vi "LV SciSDK INIT TOF SPECTRUM.vi"(0 "TOF Spectrum Name":string, 5 "Bin Width":u32, 7 "Start Delay":u32, 9 "Handle In":T2, 11 "error in (no error)":errorcluster) -> (10 "TOF Spectrum Handle Out":T1, 15 "error out":errorcluster)   [LabVIEW 2021]
uses:
  SciSDK_Labview.lvlib
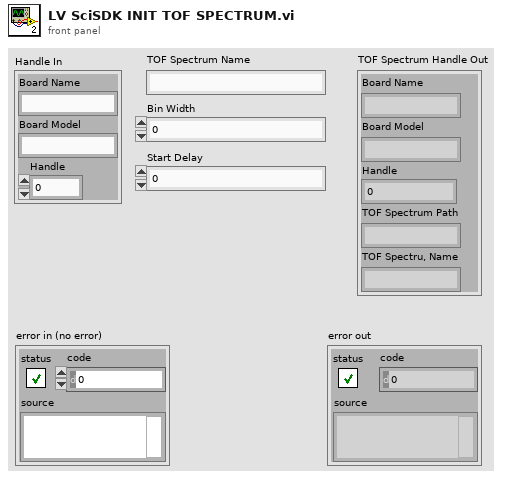
[diagram p1: front panel]
types:
  T1 = cluster{"Board Name":string, "Board Model":string, "Handle":u64, "TOF Spectrum Path":string, "TOF Spectru, Name":string}
  T2 = cluster{"Board Name":string, "Board Model":string, "Handle":u64}
  T3 = cluster{"Board Name":string, "Board Model":string, "Handle":u64, string, "TOF Spectrum Name":string}
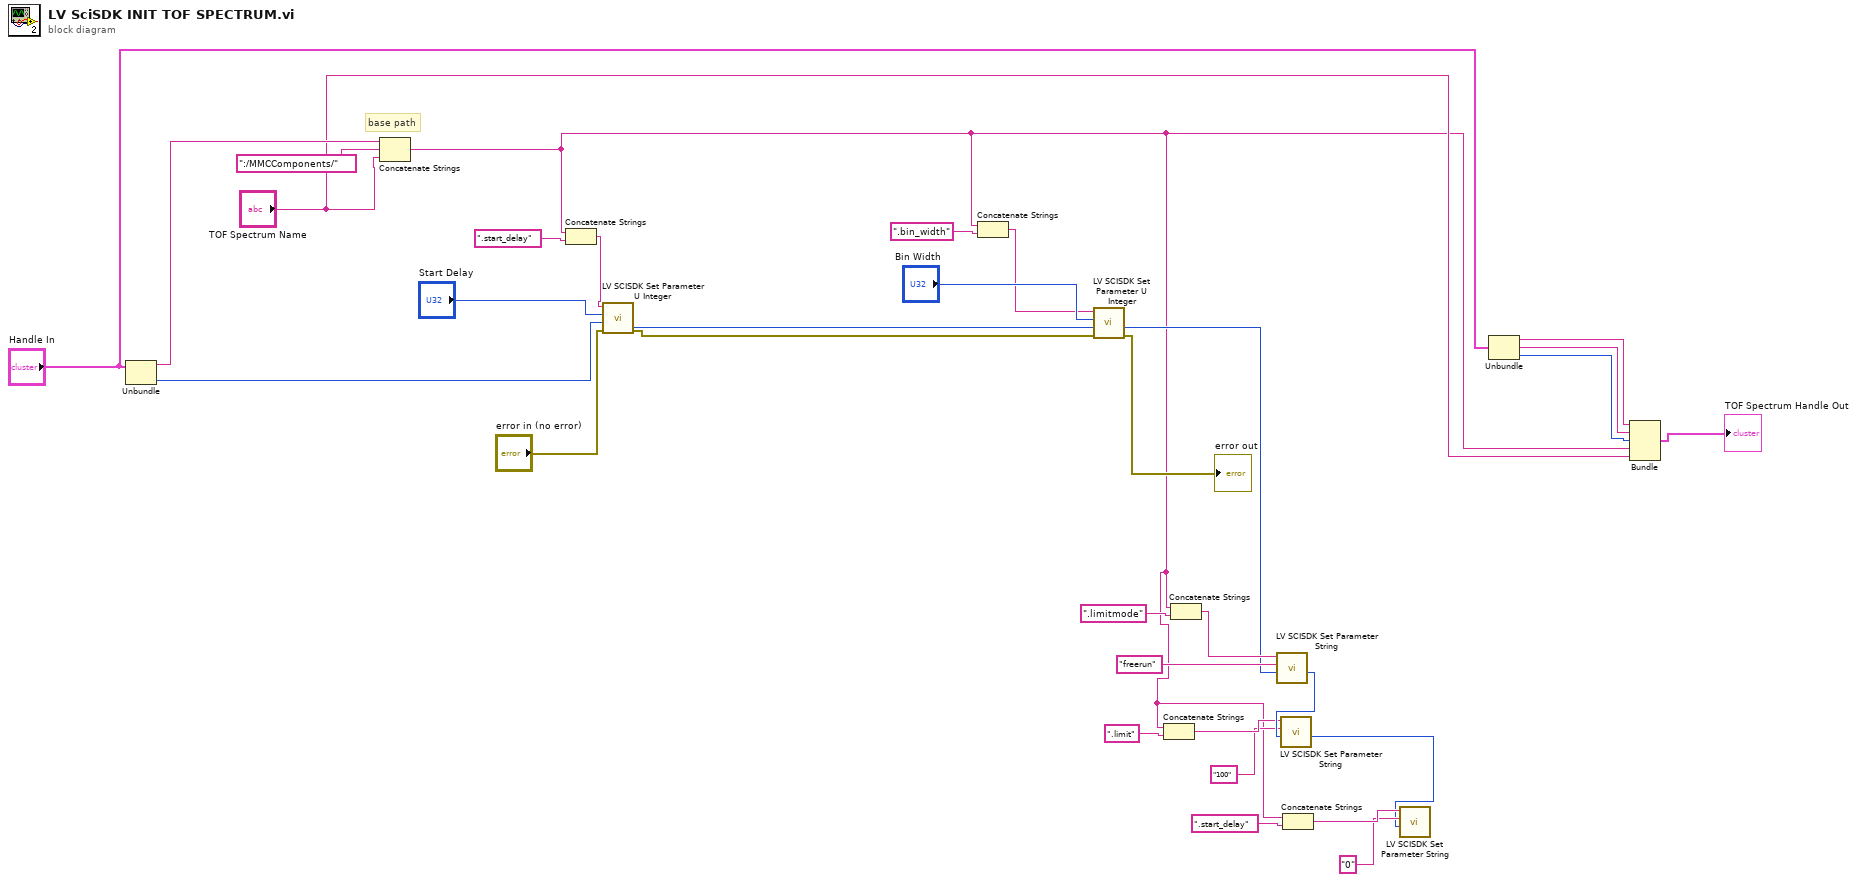
[diagram p0: block diagram]
diagram:
  # "base path"
  n1 = Unbundle("Handle In") -> ("Board Name"=w31:string, "Handle"=w17:u64)  [unwired: 1 out]
  n2 = Concatenate Strings(w31, ":/MMCComponents/" ("string"), "TOF Spectrum Name") -> (w1:string)
  n3 = Concatenate Strings(w1, ".start_delay" ("string")) -> (w20:string)
  n4 = call "LV SCISDK Set Parameter U Integer.vi"("error in (no error)"="error in (no error)", "handle"=w17, "value"="Start Delay", "Path"=w20) -> ("error out"=w14:errorcluster, "handle out"=w18:u64)  [unwired: 5 in, 1 out]
  n5 = Concatenate Strings(w1, ".bin_width" ("string")) -> (w19:string)
  n6 = call "LV SCISDK Set Parameter U Integer.vi"("error in (no error)"=w14, "handle"=w18, "value"="Bin Width", "Path"=w19) -> ("error out"=→"error out":errorcluster, "handle out"=w10:u64)  [unwired: 5 in, 1 out]
  n7 = Concatenate Strings(w1, ".limit" ("string")) -> (w7:string)
  n8 = Concatenate Strings(w1, ".limitmode" ("string")) -> (w12:string)
  n9 = call "LV SCISDK Set Parameter String.vi"("handle"=w10, "value"="freerun", "Path"=w12) -> ("handle out"=w9:u64)  [unwired: 6 in, 2 out]
  n10 = call "LV SCISDK Set Parameter String.vi"("handle"=w9, "value"="100", "Path"=w7) -> ("handle out"=w2:u64)  [unwired: 6 in, 2 out]
  n11 = Concatenate Strings(w1, ".start_delay" ("string")) -> (w4:string)
  n12 = call "LV SCISDK Set Parameter String.vi"("handle"=w2, "value"="0", "Path"=w4) -> ()  [unwired: 6 in, 3 out]
  n13 = Unbundle("Handle In") -> ("Board Name"=w27:string, "Board Model"=w26:string, "Handle"=w25:u64)
  n14 = Bundle("Board Name"=w27, "Board Model"=w26, "Handle"=w25, w1, "TOF Spectrum Name"="TOF Spectrum Name") -> (→"TOF Spectrum Handle Out":T3)  [unwired: 1 in]
